vi "Close.vi"(8 "error in":errorcluster, 9 "timeout (-1)":i32=-1, 11 "Engine Runtime Interface in":refnum<class "Engine Runtime Interface.lvclass">) -> (0 "error out":errorcluster)   [LabVIEW 2014, in "Engine Runtime Interface.lvclass"]
doc: "Cleans up and closes an engine that was previously opened."
uses:
  Engine Runtime Interface.lvclass
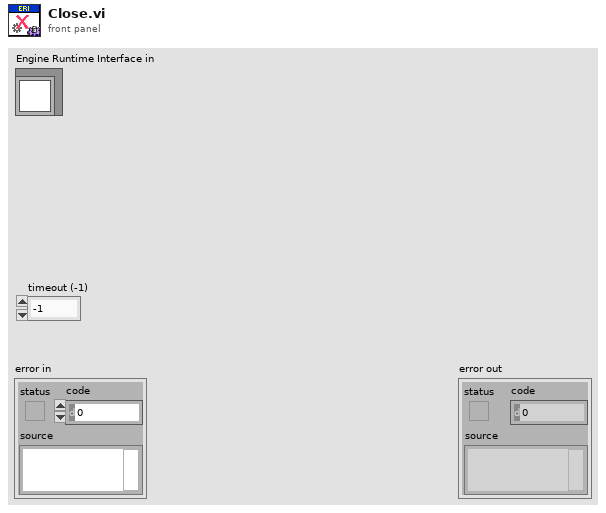
[diagram p1: front panel]
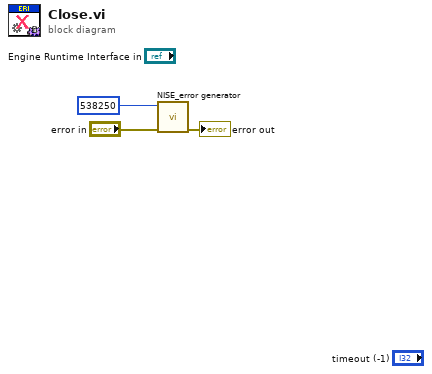
[diagram p0: block diagram]
diagram:
  n1 = call <vilib>:"NISE_error generator.vi"("error in"="error in", "error code (0)"=538250) -> ("error out"=→"error out":errorcluster)  [unwired: 7 in]
